vi "4-wire-post-logic.vi"(9 "Ready For Output in":bool, 10 "register state in":bool, 11 "output valid in":bool) -> (2 "ready for input out":bool, 3 "output valid out":bool)   [LabVIEW 2018, in "SCTL.lvlib"]
uses:
  SCTL.lvlib
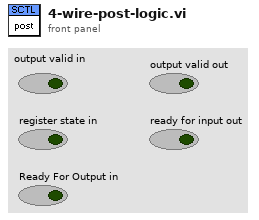
[diagram p1: front panel]
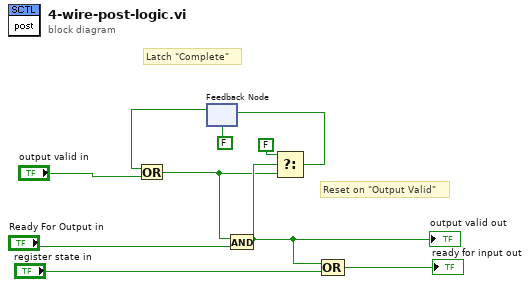
[diagram p0: block diagram]
diagram:
  # "Reset on \"Output Valid\""
  # "Latch \"Complete\""
  n1 = feedback #1(FALSE ("x .and. y?")) -> (w6:bool)
  n2 = Or(x=w6, y="output valid in") -> (x .or. y?=w4:bool)
  n3 = And(x=w4, y="Ready For Output in") -> (x .and. y?=w10:bool)
  "output valid out" <- w10
  n4 = Select(t=FALSE, s=w10, f=w4) -> (s? t:f=w5:bool)
  n5 = feedback-in #1(w5) -> ()
  n6 = Compound Arithmetic op=OR(w10, "register state in") -> (→"ready for input out":bool)
